vi "Main Process Case All.vi"(11 "Main Process Class In":refnum<class "Main Class.lvclass">) -> (0 "error out":errorcluster, 1 "KeepCase":bool)   [LabVIEW 2019]
uses:
  Class/Main Process Class/Main Class.lvclass
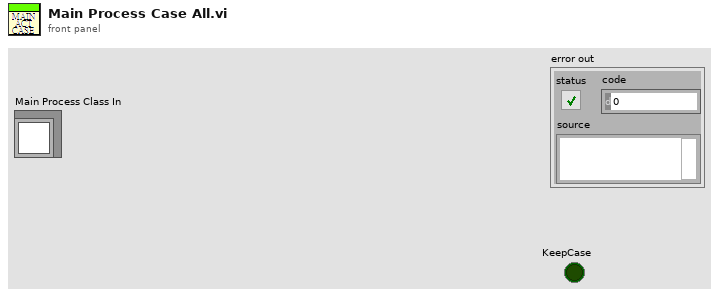
[diagram p1: front panel]
types:
  T1 = enum16{"Initial", "Add", "Read", "Delete & Check"}
  T2 = cluster{"AutoRunFlg":refnum<vi>, "Action Finish Flg":refnum<vi>, "Remaining Action":refnum<vi>, "Btn_AutoRun":refnum<vi>, "Manual Flg":refnum<vi>, "Sub Process Error":refnum<vi>}
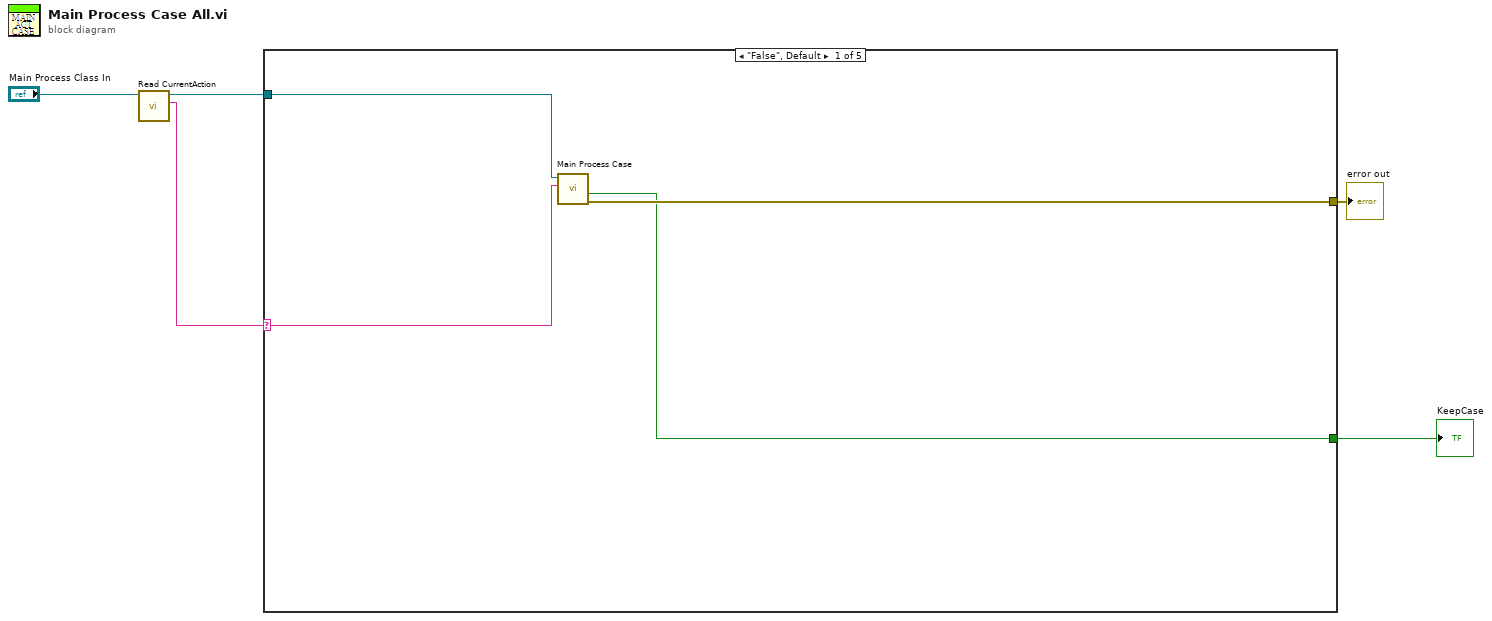
[diagram p0: block diagram]
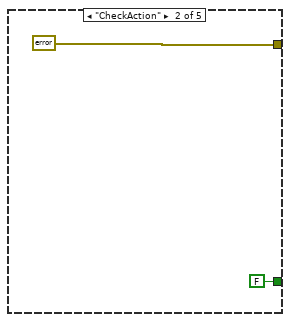
[diagram p2: hidden frame]
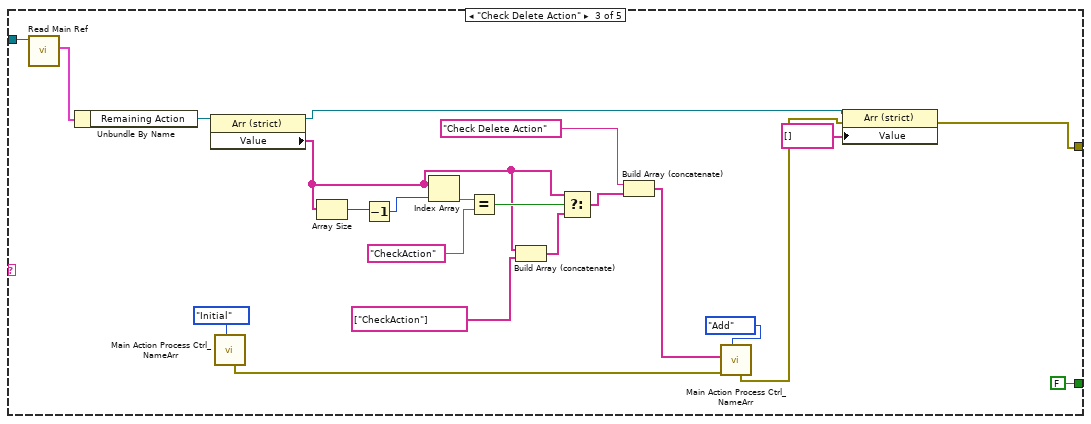
[diagram p3: hidden frame]
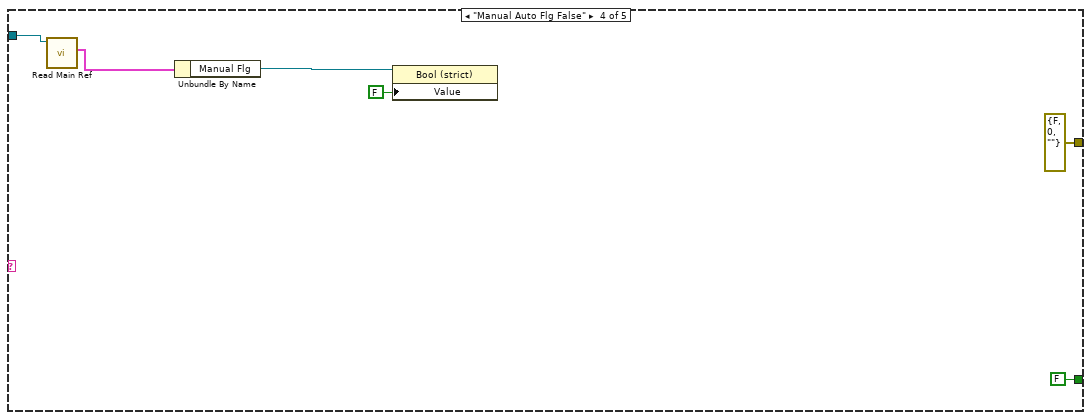
[diagram p4: hidden frame]
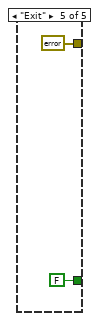
[diagram p5: hidden frame]
diagram:
  n1 = call-dynamic "Read CurrentAction.vi"("Main Process Class in"="Main Process Class In") -> ("CurrentAction"=w1:string, "Main Process Class out"=w2:refnum<class "Main Class.lvclass">)  [unwired: 8 in, 1 out]
  n2 = case shown="\"False\", Default" w1 {
    selector: w1 -> [w6 _ _ _ _]
    tunnel: w2 -> [w9 _ w32 w39 _]
    tunnel: [w8 errorcluster {"status"=FALSE, "code"=0, "source"=""} ("error out") w12 errorcluster {"status"=FALSE, "code"=0, "source"=""} ("error out") errorcluster {"status"=FALSE, "code"=0, "source"=""} ("error out")] -> w4
    tunnel: [w7 FALSE ("delete case") FALSE ("delete case") FALSE ("delete case") FALSE ("delete case")] -> w3
    frame "False", Default {
      n3 = call-dynamic "Main Process Case.vi"("CurrentAction"=w6, "Main Process Class in"=w9) -> ("error out"=w8:errorcluster, "KeepCase"=w7:bool)  [unwired: 7 in, 1 out]
    }
    frame "CheckAction" {
    }
    frame "Check Delete Action" {
      n4 = call-dynamic "Read Main Ref.vi"("Main Process Class in"=w32) -> ("Main Ref"=w31:T2)  [unwired: 8 in, 2 out]
      n5 = Unbundle By Name(w31) -> ("Remaining Action"=w30:refnum<vi>)
      n6 = property class="Arr (strict)"(reference=w30) -> (reference out=w15:refnum<vi>, "Value"=w23:string[])  [unwired: 1 in, 1 out]
      n7 = call "Main Action Process Ctrl_NameArr.vi"("Action"=T1."Initial") -> ("error out"=w19:errorcluster)  [unwired: 6 in, 4 out]
      n8 = Array Size(array=w23) -> (size(s)=w29:i32)
      n9 = Decrement(x=w29) -> (x-1=w28:i32)
      n10 = Index Array(array=w23, index=w28) -> (element=w27:string)
      n11 = Equal?(x=w27, y="CheckAction") -> (x = y?=w26:bool)
      n12 = Build Array (concatenate)(w23, string[] ["CheckAction"]) -> (w22:string[])
      n13 = Select(t=w23, s=w26, f=w22) -> (s? t:f=w18:string[])
      n14 = Build Array (concatenate)("Check Delete Action" ("y"), w18) -> (w16:string[])
      n15 = call "Main Action Process Ctrl_NameArr.vi"("Action"=T1."Add", "error in"=w19, "Add Action Que"=w16) -> ("error out"=w13:errorcluster)  [unwired: 4 in, 4 out]
      n16 = property class="Arr (strict)"(reference=w15, error in=w13, "Value"=string[] []) -> (error out=w12:errorcluster)  [unwired: 1 out]
    }
    frame "Manual Auto Flg False" {
      n17 = call-dynamic "Read Main Ref.vi"("Main Process Class in"=w39) -> ("Main Ref"=w38:T2)  [unwired: 8 in, 2 out]
      n18 = Unbundle By Name(w38) -> ("Manual Flg"=w37:refnum<vi>)
      n19 = property class="Bool (strict)"(reference=w37, "Value"=FALSE) -> ()  [unwired: 1 in, 2 out]
    }
    frame "Exit" {
    }
  }
  "error out" <- w4
  "KeepCase" <- w3
